vi "Thingworx_ReadAll.vi"(8 "error in (no error)":errorcluster, 10 "Thing":string, 11 "Device in":T2) -> (0 "error out":errorcluster, 2 "Properties":string[][](table)=[["test", "test", "STRING"]], 3 "Device Out":T2)   [LabVIEW 2016]
uses:
  _subVIs/Device.ctl
  _subVIs/HTTPComm.ctl
panel:
  out "Comm":T1
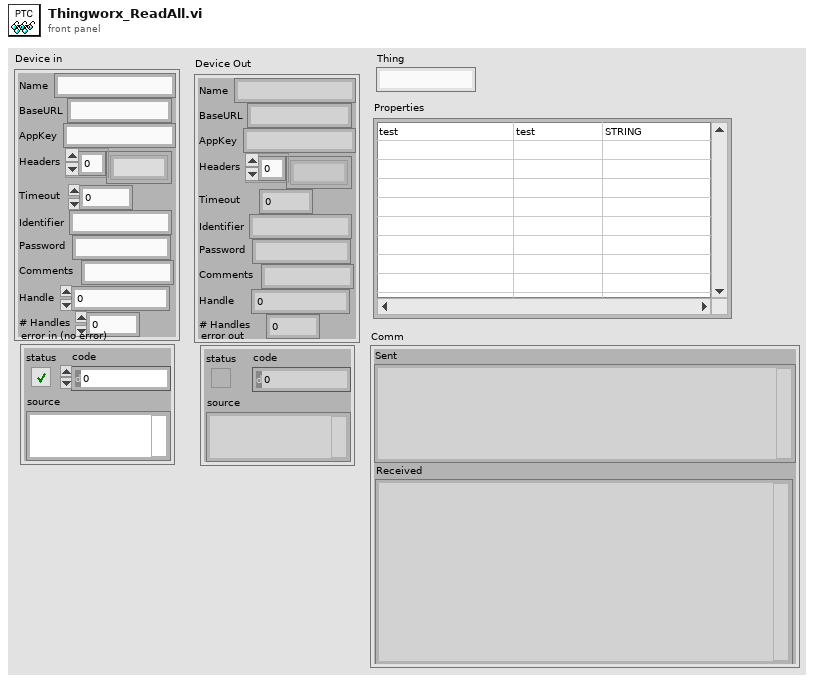
[diagram p1: front panel]
types:
  T1 = typedef "HTTPComm.ctl" = cluster{"url":string, "sent headers":string, "sent body":string, "headers":string, "body":string, "Sent":string, "Received":string}
  T2 = typedef "Device.ctl" = cluster{"Name":string, "BaseURL":string, "AppKey":string, "Headers":string[], "Timeout":i32, "Identifier":string, "Password":string, "Comments":string, "Handle":u32, "# Handles":i32}
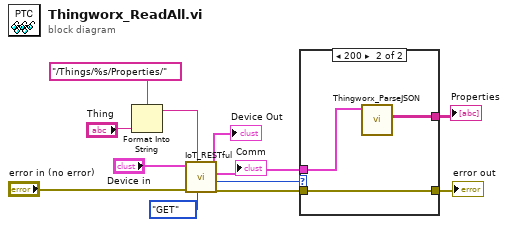
[diagram p0: block diagram]
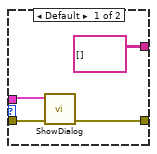
[diagram p2: hidden frame]
diagram:
  n1 = Format Into String(format string="/Things/%s/Properties/", "Thing") -> (resulting string=w10:string)  [unwired: 2 in, 1 out]
  n2 = call "IoT_RESTful.vi"("Method"=enum16{"GET", "PUT", "POST", "MultiPOST"}."GET", "url"=w10, "error in"="error in (no error)", "Device In"="Device in") -> ("error out"=w12:errorcluster, "HTTP Code"=w11:i32, "Comm"=w7:T1, "Device Out"=→"Device Out":T2)  [unwired: 4 in]
  "Comm" <- w7
  n3 = case shown="200" w11 {
    tunnel: w7 -> [w14 w18]
    tunnel: w12 -> [w15 w16]
    tunnel: [w15 w16] -> w1
    tunnel: [string[][] [] ("Table Control") w17] -> w2
    frame Default {
      n4 = call "ShowDialog.vi"("Comm"=w14) -> ()  [unwired: 11 in]
    }
    frame 200 {
      n5 = call "Thingworx_ParseJSON.vi"("Comm"=w18) -> ("Table Control"=w17:string[][])  [unwired: 9 in, 1 out]
    }
  }
  "Properties" <- w2
  "error out" <- w1
